vi "e.gate HighSpeedPort Read Buffer Header.vi"(8 "error in (no error)":errorcluster, 11 "Configuration in":T1) -> (0 "error out":errorcluster, 3 "Configuration out":T1)   [LabVIEW 2016]
doc: "This VI is used to receive and decode buffer header data to the configuration cluster."
uses:
  e.gate Configuration.ctl
  e.gate Channel Data.ctl
  e.gate Data Type.ctl
  e.gate Protocol Type.ctl
  e.gate Module  Data.ctl
  e.gateHSP_DLLhandle.ctl
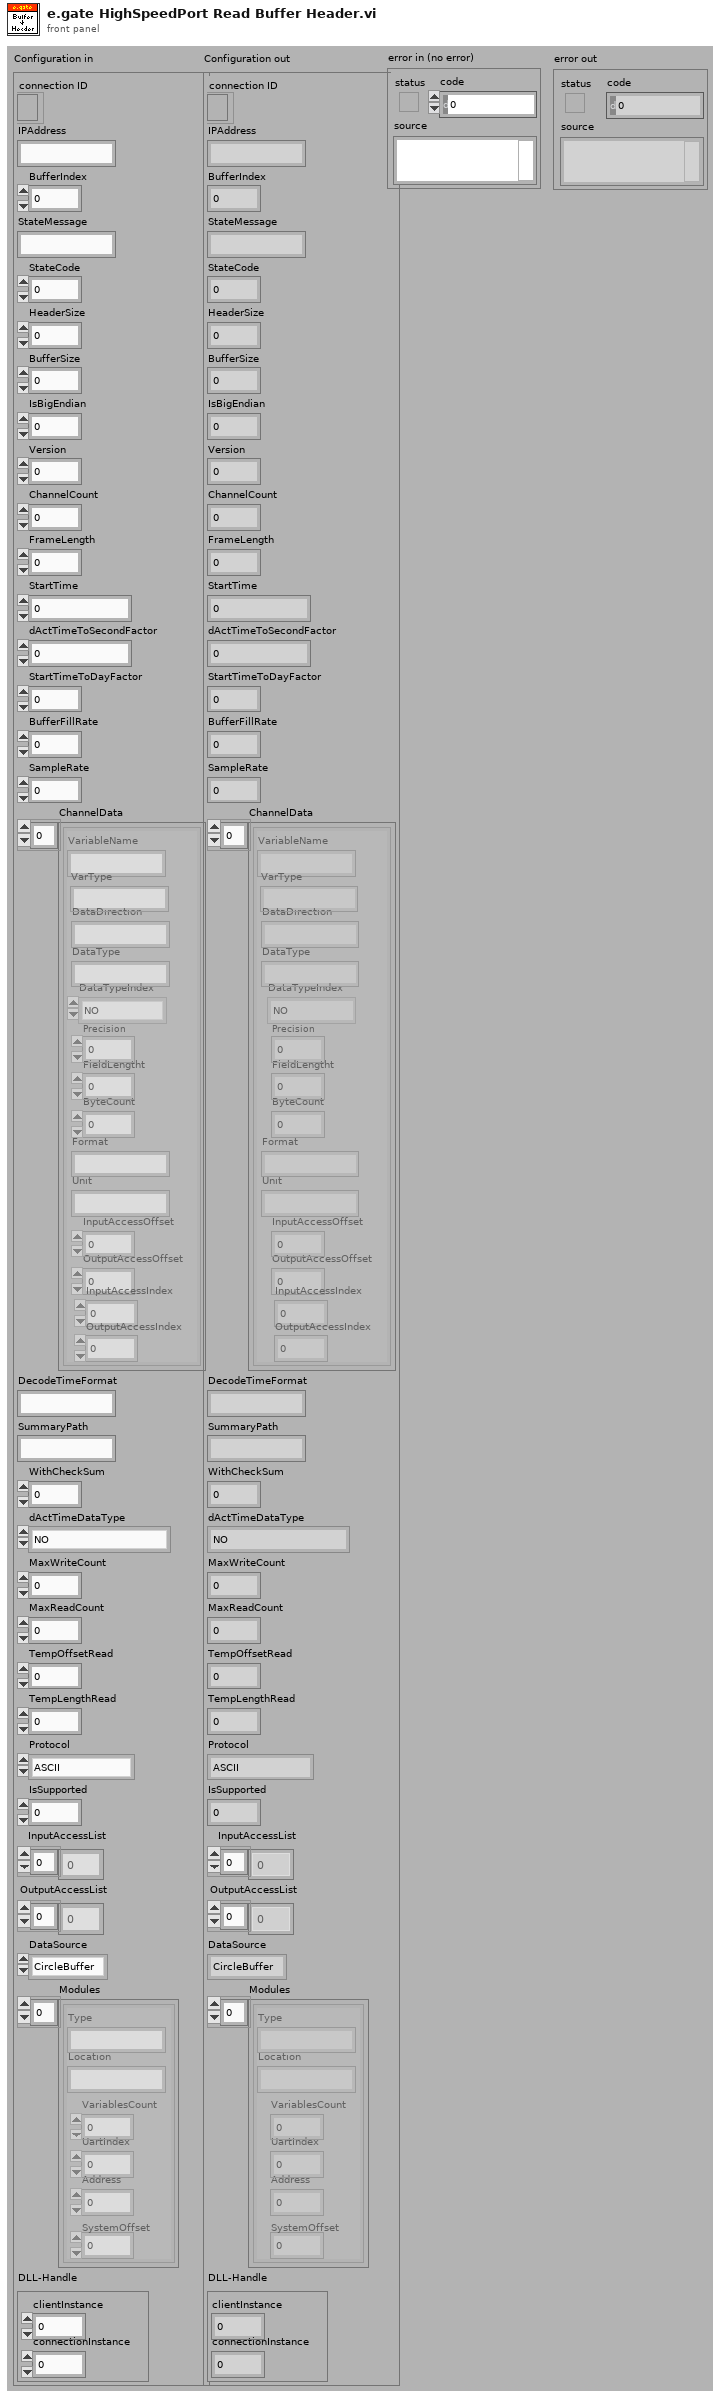
[diagram p1: front panel]
types:
  T1 = typedef "e.gate Configuration.ctl" = cluster{"connection ID":refnum<k5>, "IPAddress":string, "BufferIndex":i32, "StateMessage":string, "StateCode":i8, "HeaderSize":i32, "BufferSize":i32, "IsBigEndian":i32, "Version":i32, "ChannelCount":i32, "FrameLength":i32, "StartTime":dbl, "dActTimeToSecondFactor":dbl, "StartTimeToDayFactor":dbl, "BufferFillRate":dbl, "SampleRate":dbl, "ChannelData":T2[], "DecodeTimeFormat":string, "SummaryPath":string, "WithCheckSum":i32, "dActTimeDataType":T3, "MaxWriteCount":i32, "MaxReadCount":i32, "TempOffsetRead":i32, "TempLengthRead":i32, "Protocol":T4, "IsSupported":i32, "InputAccessList":i32[], "OutputAccessList":i32[], "DataSource":enum16{"CircleBuffer", "test.con Logger", "test.con Archive"}, "Modules":T5[], "DLL-Handle":T6}
  T2 = typedef "e.gate Channel Data.ctl" = cluster{"VariableName":string, "DataDirection":string, "DataType":string, "DataTypeIndex":T3, "Precision":i16, "FieldLengtht":i16, "ByteCount":i32, "Format":string, "Unit":string, "InputAccessOffset":i32, "OutputAccessOffset":i16, "InputAccessIndex":i16, "OutputAccessIndex":i16, "VarType":string}
  T3 = typedef "e.gate Data Type.ctl" = enum16{"NO", "BOOL", "SINT8", "USINT8", "SINT16", "USINT16", "SINT32", "USINT32", "FLOAT", "SET8", "SET16", "SET32", "DOUBLE", "SINT64", "USINT64", "SET64"}
  T4 = typedef "e.gate Protocol Type.ctl" = enum16{"ASCII", "HighspeedPort Online", "HighspeedPort Buffer", "eGateHighspeedPortDLL "}
  T5 = typedef "e.gate Module  Data.ctl" = cluster{"Type":string, "Location":string, "VariablesCount":i16, "UartIndex":i16, "Address":i16, "SystemOffset":i16}
  T6 = typedef "e.gateHSP_DLLhandle.ctl" = cluster{"clientInstance":i32, "connectionInstance":i32}
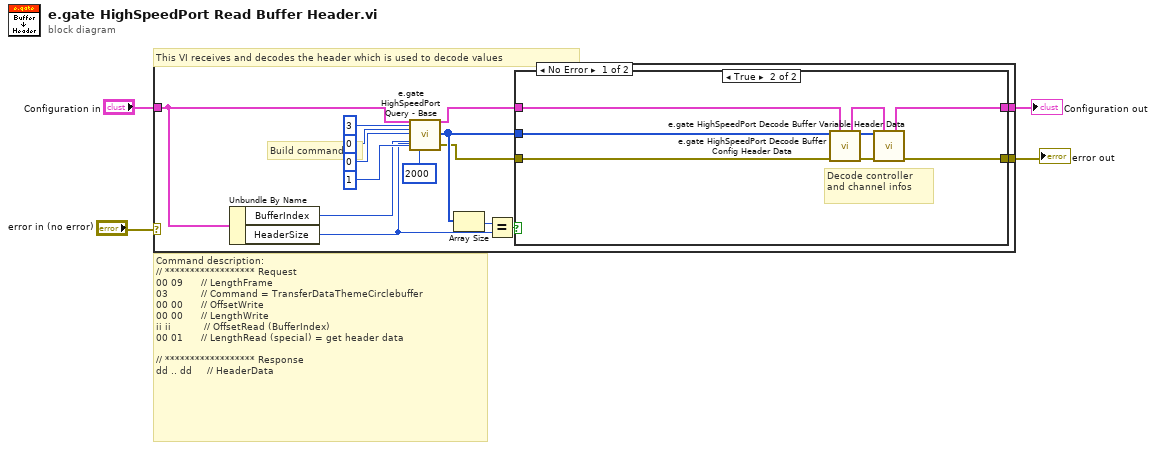
[diagram p0: block diagram]
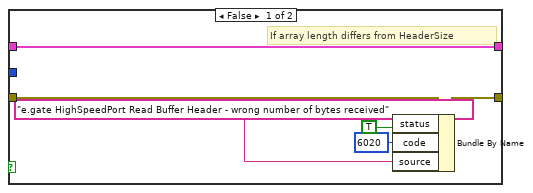
[diagram p2: hidden frame]
diagram:
  # "This VI receives and decodes the header which is used to decode values"
  # "Command description:\n// ****************** Request\n00 09\t\t\t\t\t\t// LengthFrame\n03\t\t\t\t\t\t    \t// Command = TransferDataThemeCirclebuffer\n00 00\t\t\t\t\t\t// OffsetWrite\n00 00\t\t\t\t\t\t// LengthWrite\nii ii\t\t\t\t\t     \t// OffsetRead (BufferIndex)\n00 01\t\t\t\t\t\t// LengthRead (special) = get header data\n\n// ****************** Response\ndd .. dd\t\t\t\t\t// HeaderData"
  n1 = case shown="No Error" "error in (no error)" {
    selector: "error in (no error)" -> [_ w34]
    tunnel: "Configuration in" -> [w6 w35]
    tunnel: [w9 w35] -> w4
    tunnel: [w8 w34] -> w1
    frame No Error {
      # "Build command"
      n2 = Unbundle By Name(w6) -> ("BufferIndex"=w14:i32, "HeaderSize"=w12:i32)
      n3 = call "e.gate HighSpeedPort Query - Base.vi"("e.gate Configuration in"=w6, "Command"=3, "OffsetWrite"=0 ("Command"), "LengthWrite"=0 ("Command"), "OffsetRead"=w14, "LengthRead"=1 ("Command"), "TCP LengthReadt"=w12, "Timeout (1000)"=2000) -> ("e.gate Configuration out"=w5:T1, "Data (out binary)"=w11:u8[], "error out"=w10:errorcluster)  [unwired: 2 in, 15 out]
      n4 = Array Size(array=w11) -> (size(s)=w13:i32)
      n5 = Equal?(x=w13, y=w12) -> (x = y?=w7:bool)
      n6 = case shown="True" w7 {
        tunnel: w11 -> [_ w33]
        tunnel: w10 -> [w24 w32]
        tunnel: w5 -> [w25 w31]
        tunnel: [w25 w27] -> w9
        tunnel: [w23 w26] -> w8
        frame False {
          # "If array length differs from HeaderSize"
          n7 = Bundle By Name(cluster=w24, "status"=TRUE, "code"=6020, "source"="e.gate HighSpeedPort Read Buffer Header - wrong number of bytes received") -> (w23:errorcluster)
        }
        frame True {
          # "Decode controller\nand channel infos"
          n8 = call "e.gate HighSpeedPort Decode Buffer Config Header Data.vi"("Data in (binary)"=w33, "Configuration in"=w31, "error in (no error)"=w32) -> ("Configuration out"=w30:T1, "Data out (binary)"=w29:u8[], "error out"=w28:errorcluster)  [unwired: 10 out]
          n9 = call "e.gate HighSpeedPort Decode Buffer Variable Header Data.vi"("Data in (binary)"=w29, "Configuration in"=w30, "error in (no error)"=w28) -> ("Configuration out"=w27:T1, "error out"=w26:errorcluster)  [unwired: 11 out]
        }
      }
    }
    frame Error {
    }
  }
  "Configuration out" <- w4
  "error out" <- w1
